vi "Init.vi"(3 "Container State":T5, 4 "Previous State":variant, 5 "Previous Version":T4) -> (2 "Current State":T2)   [LabVIEW 2020, in "Waveform (G3).xctl"]
uses:
  Waveform (G3).xctl
  State.ctl
  Utility VIs/Controls/KRing/KRing.xctl
  Tone (G3)/Tone (G3).xctl
  Noise (G3)/Noise (G3).xctl
  Noise (G3)/Noise (G3) - Persistent.ctl
  <vilib>/_xctls/Container State.ctl
  <vilib>/_xctls/Version.ctl
  Waveform VIs/Waveform Enum (V3).ctl
  <vilib>/_xctls/XControlSupport.lvlib
panel:
  in  "Waveform":T1
  in  "Default Indicator State":T2
  in  "Default Control State":T2
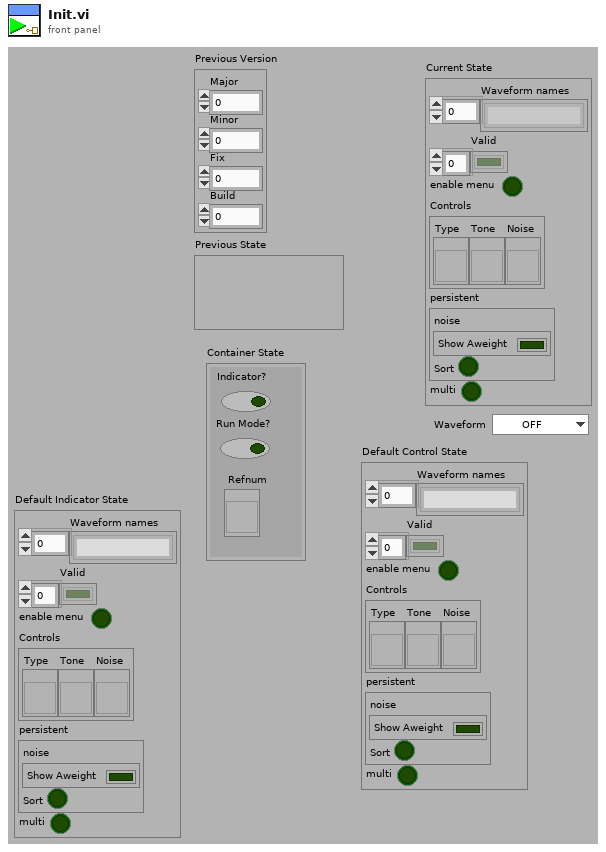
[diagram p1: front panel]
types:
  T1 = typedef "Waveform Enum (V3).ctl" = enum16{"OFF", "Tone", "Noise", "Pulse Train", "File", "FM Sweep", "Chirp Train", "Complex Tone", "FM Tone", "Vowel", "Ramp"}
  T2 = typedef "Waveform (G3).xctl/State.ctl" = cluster{"Waveform names":string[], "Valid":bool[], "enable menu":bool, "Controls":cluster{"Type ":refnum<vi>, "Tone ":refnum<vi>, "Noise":refnum<vi>}, "persistent":cluster{"noise":T3, "Sort":bool}, "multi":bool}
  T3 = typedef "Noise (G3).xctl/Noise (G3) - Persistent.ctl" = cluster{"Show Aweight":bool}
  T4 = typedef "XControlSupport.lvlib/Version.ctl" = cluster{"Major":u16, "Minor":u16, "Fix":u16, "Build":u16}
  T5 = typedef "XControlSupport.lvlib/Container State.ctl" = cluster{"Indicator?":bool, "Run Mode?":bool, " Refnum":refnum<vi>}
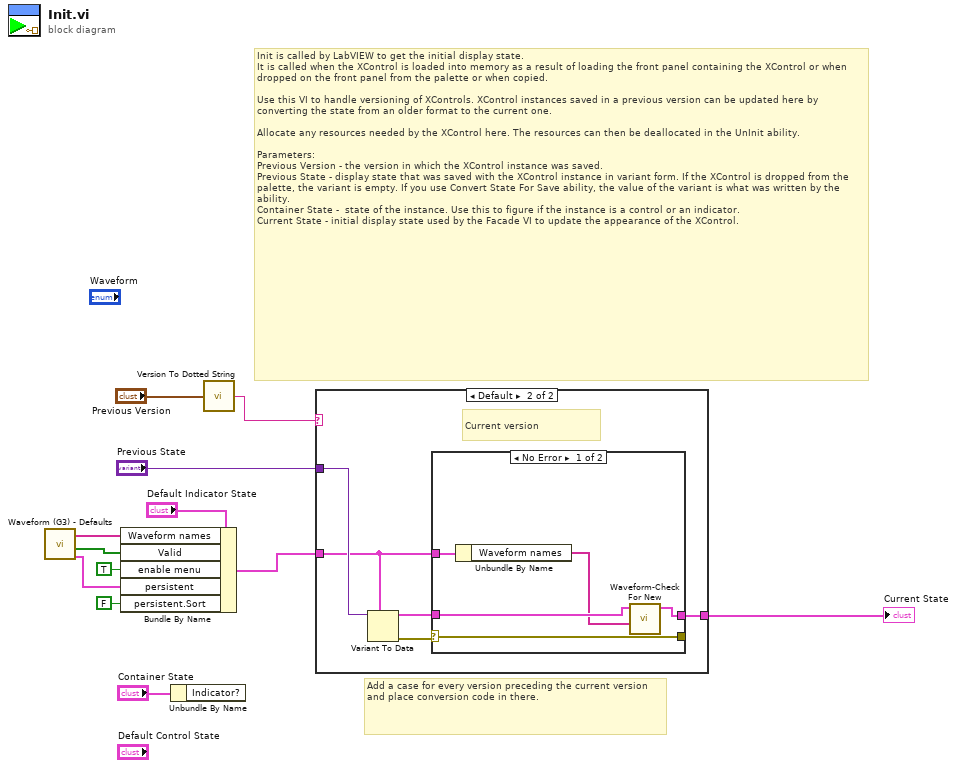
[diagram p0: block diagram]
diagram:
  # "Add a case for every version preceding the current version and place conversion code in there."
  # "Init is called by LabVIEW to get the initial display state.\nIt is called when the XControl is loaded into memory as a result of loading the front panel containing the XControl or when dropped on the front panel from the palette or when copied.\n\nUse this VI to handle versioning of XControls. XControl instances saved in a previous version can be updated here by converting the state from an older format to the current one.\n\nAllocate any resources needed by the XControl here. The resources can then be deallocated in the UnInit ability.\n\nParameters:\nPrevious Version - the version in which the XControl instance was saved.\nPrevious State - display state that was saved with the XControl instance in variant form. If the XControl is dropped from the palette, the variant is empty. If you use Convert State For Save ability, the value of the variant is what was written by the ability. \nContainer State -  state of the instance. Use this to figure if the instance is a control or an indicator.\nCurrent State - initial display state used by the Facade VI to update the appearance of the XControl."
  n1 = call "Waveform (G3) - Defaults.vi"() -> ("subcontrols"=w2:cluster{"persistent":T3, "sort":bool}, "mask"=w3:bool[], "names"=w5:string[])  [unwired: 8 in, 1 out]
  n2 = Bundle By Name(cluster="Default Indicator State", "Waveform names"=w5, "Valid"=w3, "enable menu"=TRUE, "persistent"=w2, "persistent.Sort"=FALSE ("Sort")) -> (w4:T2)
  n3 = Unbundle By Name("Container State") -> ()  [unwired: 1 out]
  n4 = call <vilib>:"Version To Dotted String.vi"("Version"="Previous Version") -> ("String Version"=w7:string)
  n5 = case shown="Default" w7 {
    tunnel: "Previous State" -> [_ w18]
    tunnel: [w13 w14] -> w11
    tunnel: w4 -> [w13 w15]
    frame "0.0.0.0" {
      # "Just created, use default state"
    }
    frame Default {
      # "Current version"
      n6 = Variant To Data(type=w15, Variant=w18) -> (data=w16:T2, error out=w17:errorcluster)  [unwired: 1 in]
      n7 = case shown="No Error" w17 {
        selector: w17 -> [w23 w24]
        tunnel: w16 -> [w21 _]
        tunnel: [w22 w25] -> w14
        tunnel: w15 -> [w20 w25]
        tunnel: [w23 w24] -> _
        frame No Error {
          n8 = Unbundle By Name(w20) -> ("Waveform names"=w19:string[])
          n9 = call "Waveform-Check For New.vi"("Waveform names"=w19, "State In"=w21) -> ("State Out"=w22:T2)  [unwired: 9 in]
        }
        frame Error {
          # "Error converting previously \nsaved state. Use default instead."
        }
      }
    }
  }
  "Current State" <- w11
